vi "溶解氧电极校准.vi"() -> ()   [LabVIEW 2016, in "斯坦道多参数.lvlib"]
uses:
  <vilib>/Utility/miscctls.llb/LVPointTypeDef.ctl
  <vilib>/Analysis/NI_AALBase.lvlib
panel:
  out "标液2":string="饱和标准液"
  out "标液1":string="零点标准液"
  in  "刷新按钮":bool
  out "第二点信号值":dbl
  out "第一点信号值":dbl
  out "通讯状态":string
  out "第二点校准值":dbl
  out "第一点校准值":dbl
  out "最小值":sgl format="%#.2f"
  out "最大值":sgl format="%#.2f"
  in  "校准模式":u16(ring)=1 items=["两点校准", "单点校准"]
  in  "校准停止":bool
  in  "校准启动":bool
  out "波形图表":dbl(graph) caption="历史曲线"
  out "变异系数":dbl format="%#.6f"
  out "standard deviation":dbl caption="标准差" format="%#.2f"
  out "mean":dbl caption="均值" format="%#.2f"
  out "测量读值":dbl caption="测量值" format="%#.2f"
  out "偏移值补偿":dbl caption="溶解氧偏移修正值" format="%#.2f"
  out "饱和度值":dbl format="%#.2f"
  out "提示":string
  out "气压补偿值":dbl format="%#.2f"
  out "盐度补偿值":dbl format="%#.2f"
  out "电极斜率":dbl format="%#.6f"
  out "电极零点":dbl format="%#.6f"
  # "溶解氧电极设定"
  # "%"
  # "%"
  # "ppt"
  # "hPa"
  # "请选择校准模式:"
  # "mg/L"
  # "%"
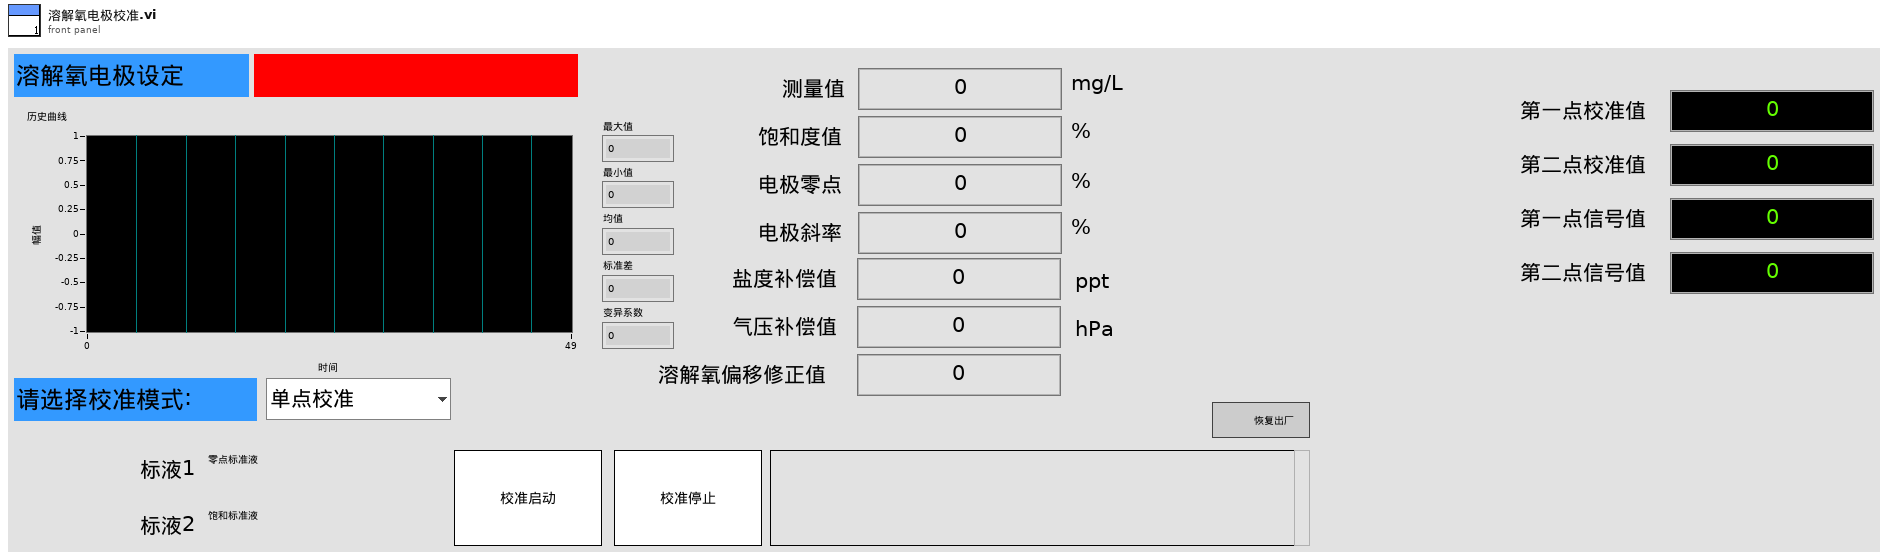
[diagram p1: front panel]
types:
  T1 = typedef "LVPointTypeDef.ctl" = cluster{"Horizontal":i16, "Vertical":i16}
  T2 = cluster{"电极状态标志":u16, "电极型号标志":u16, "溶解氧测量值":sgl, "温度测量值":sgl, "溶解氧饱和度值":sgl, "盐度补偿值":sgl, "大气压补偿值":sgl, "溶解氧偏移修正值":sgl, "温度偏移修正值":sgl, "手动温度补偿值":sgl, "溶解氧电极零点":sgl, "溶解氧电极斜率":sgl, "第1点标准值记录":sgl, "第1点信号值记录":sgl, "第1点温度值记录":sgl, "第2点标准值记录":sgl, "第2点信号值记录":sgl, "第2点温度值记录":sgl, "命令滤波设定":u16, "温度模式":enum16{"ATC", "MTC"}, "生产批次":u16, "电极序号":u16, "串口地址":u16, "串口波特率":enum16{"9600", "19200", "115200"}, "串口校验位":enum16{"NONE", "ODD", "EVEN"}, "串口停止位":enum16{"1bit", "2bit"}, "第一点标准值":sgl, "第二点标准值":sgl}
  T3 = enum8{"Enabled", "Disabled", "Disabled and Grayed Out"}
  T4 = cluster{"测量量程":dbl, "测量精度":dbl, "测量间隔":dbl, "消解温度":dbl, "消解时长":dbl, "空白校准时间":timestamp, "曲线截距":dbl, "曲线斜率":dbl, "测量检出限":dbl, "测量信号值":dbl, "线性相关系数":dbl, "二次多项式系数":dbl, "标样校准时间":timestamp, "单位":enum16{"ug/L", "mg/L"}}
  T5 = cluster{"ph":bool, "DO":bool, "Cond":bool, "Turb":bool, "叶绿素a":bool, "藻密度":bool, "ORP":bool}
  T6 = cluster{"温度测量值":sgl, "测量值":sgl, "温度偏移修正值":sgl, "信号值":sgl}
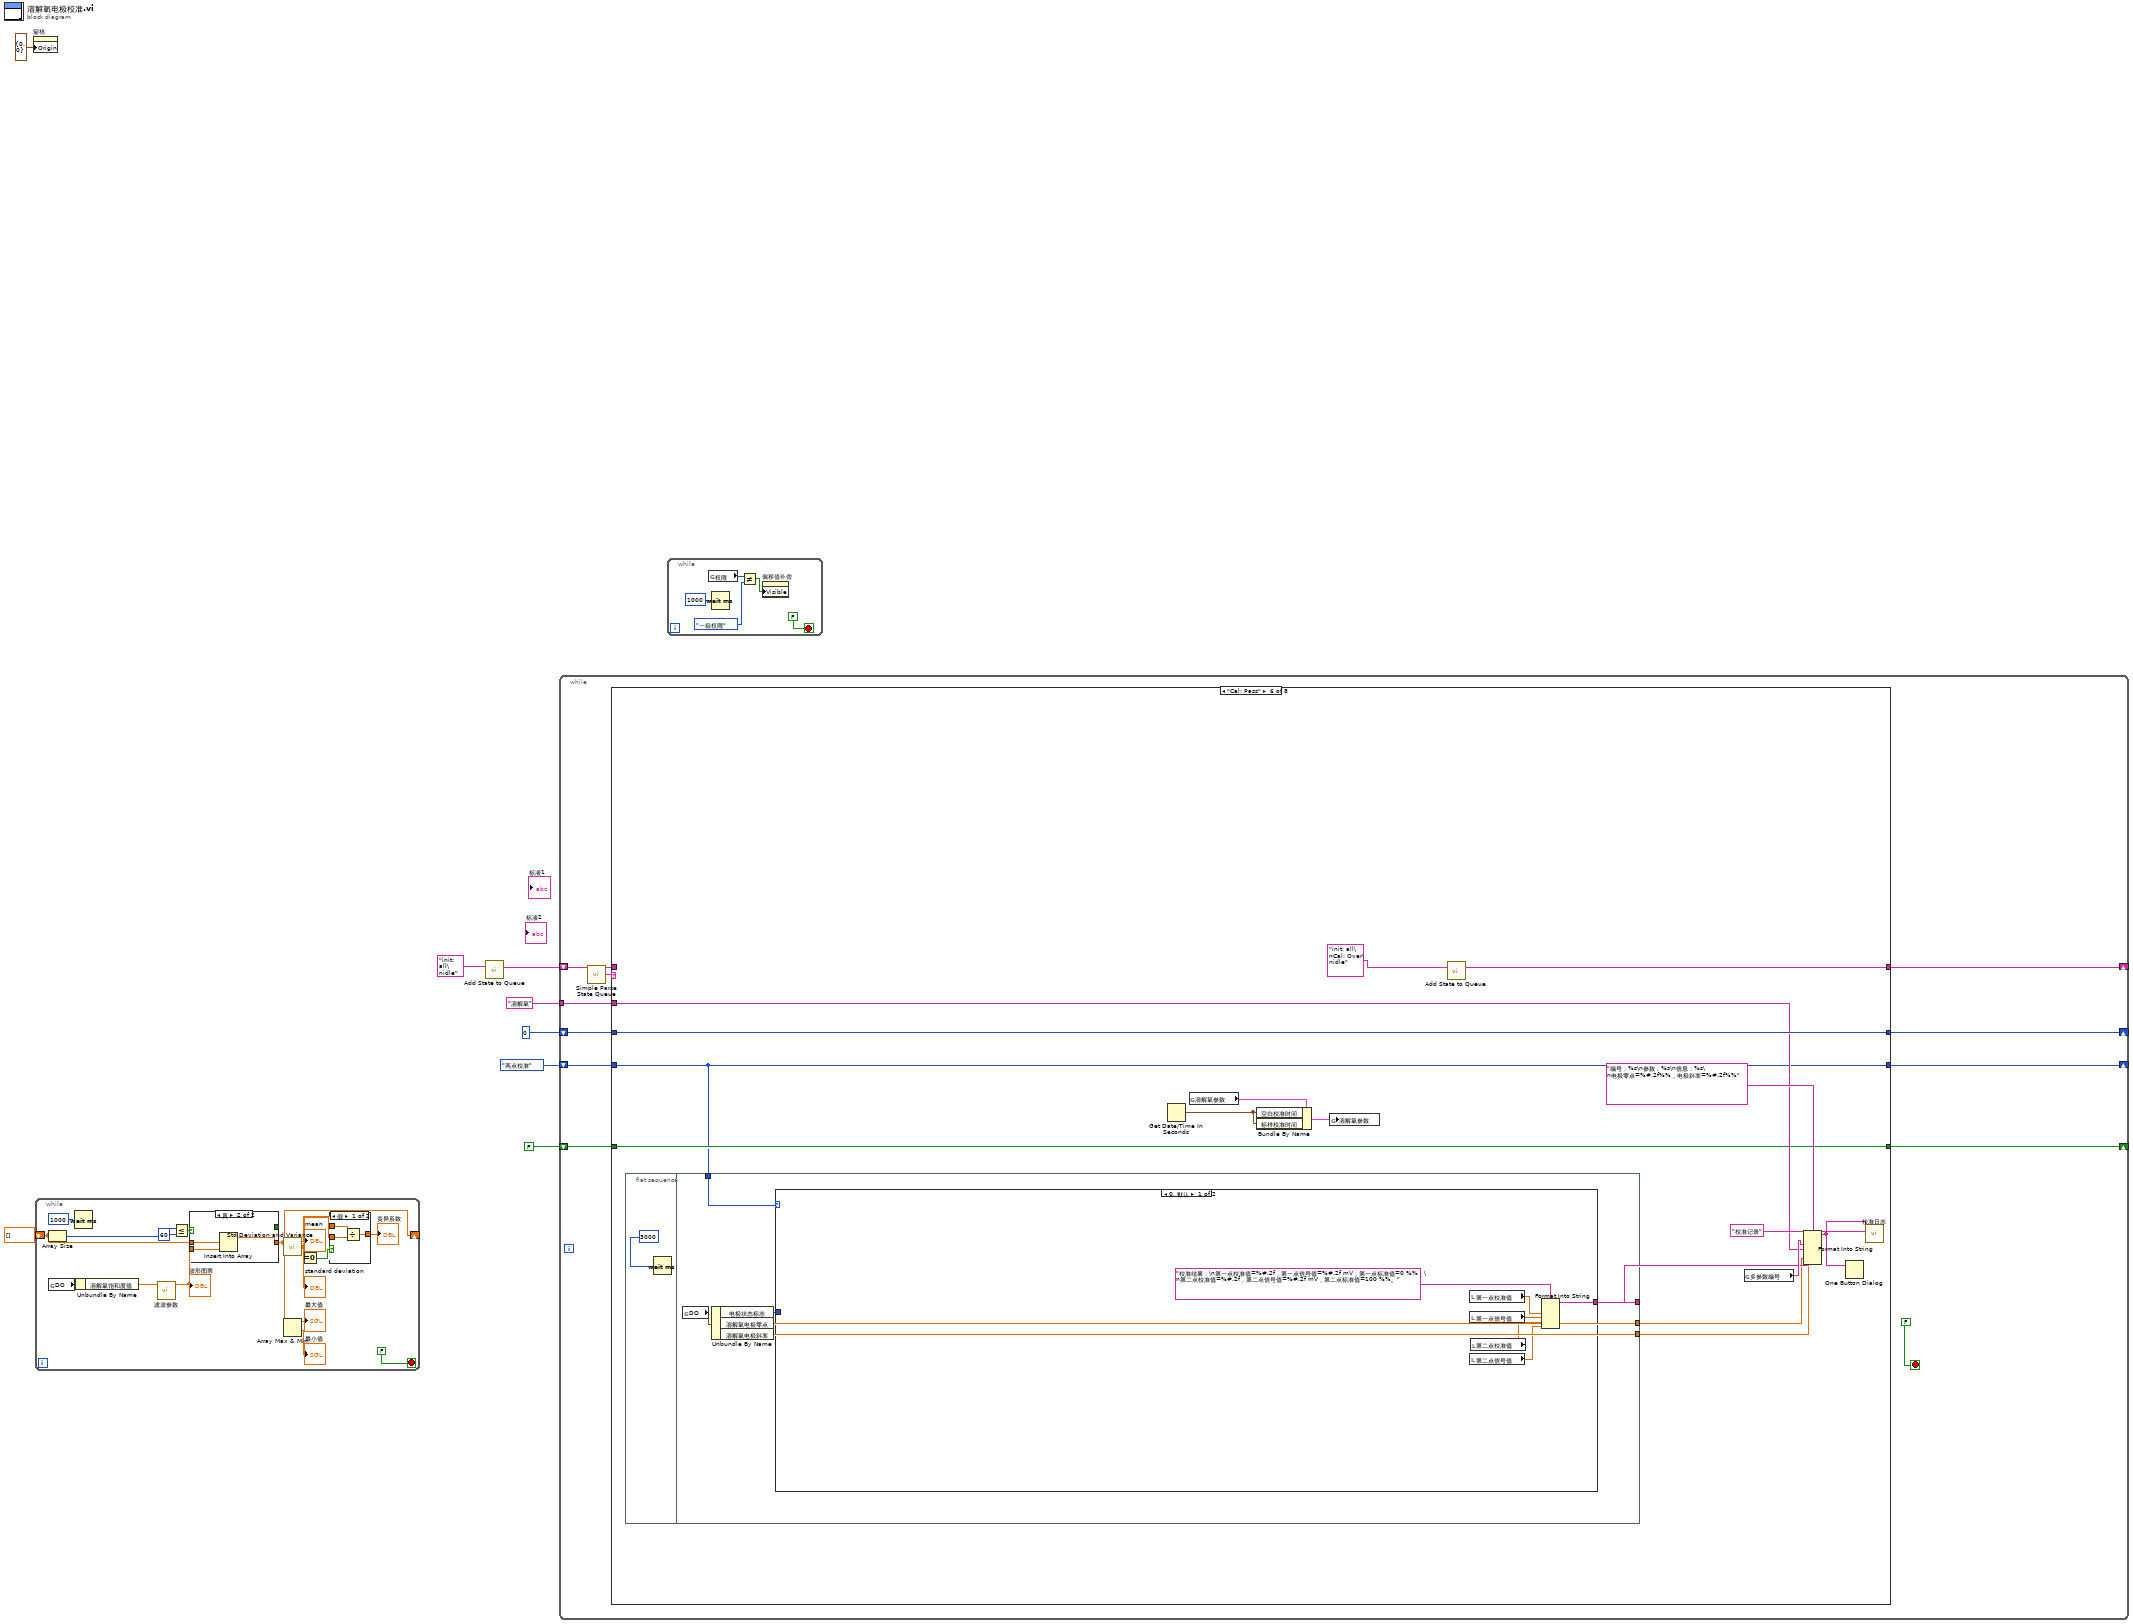
[diagram p0: block diagram]
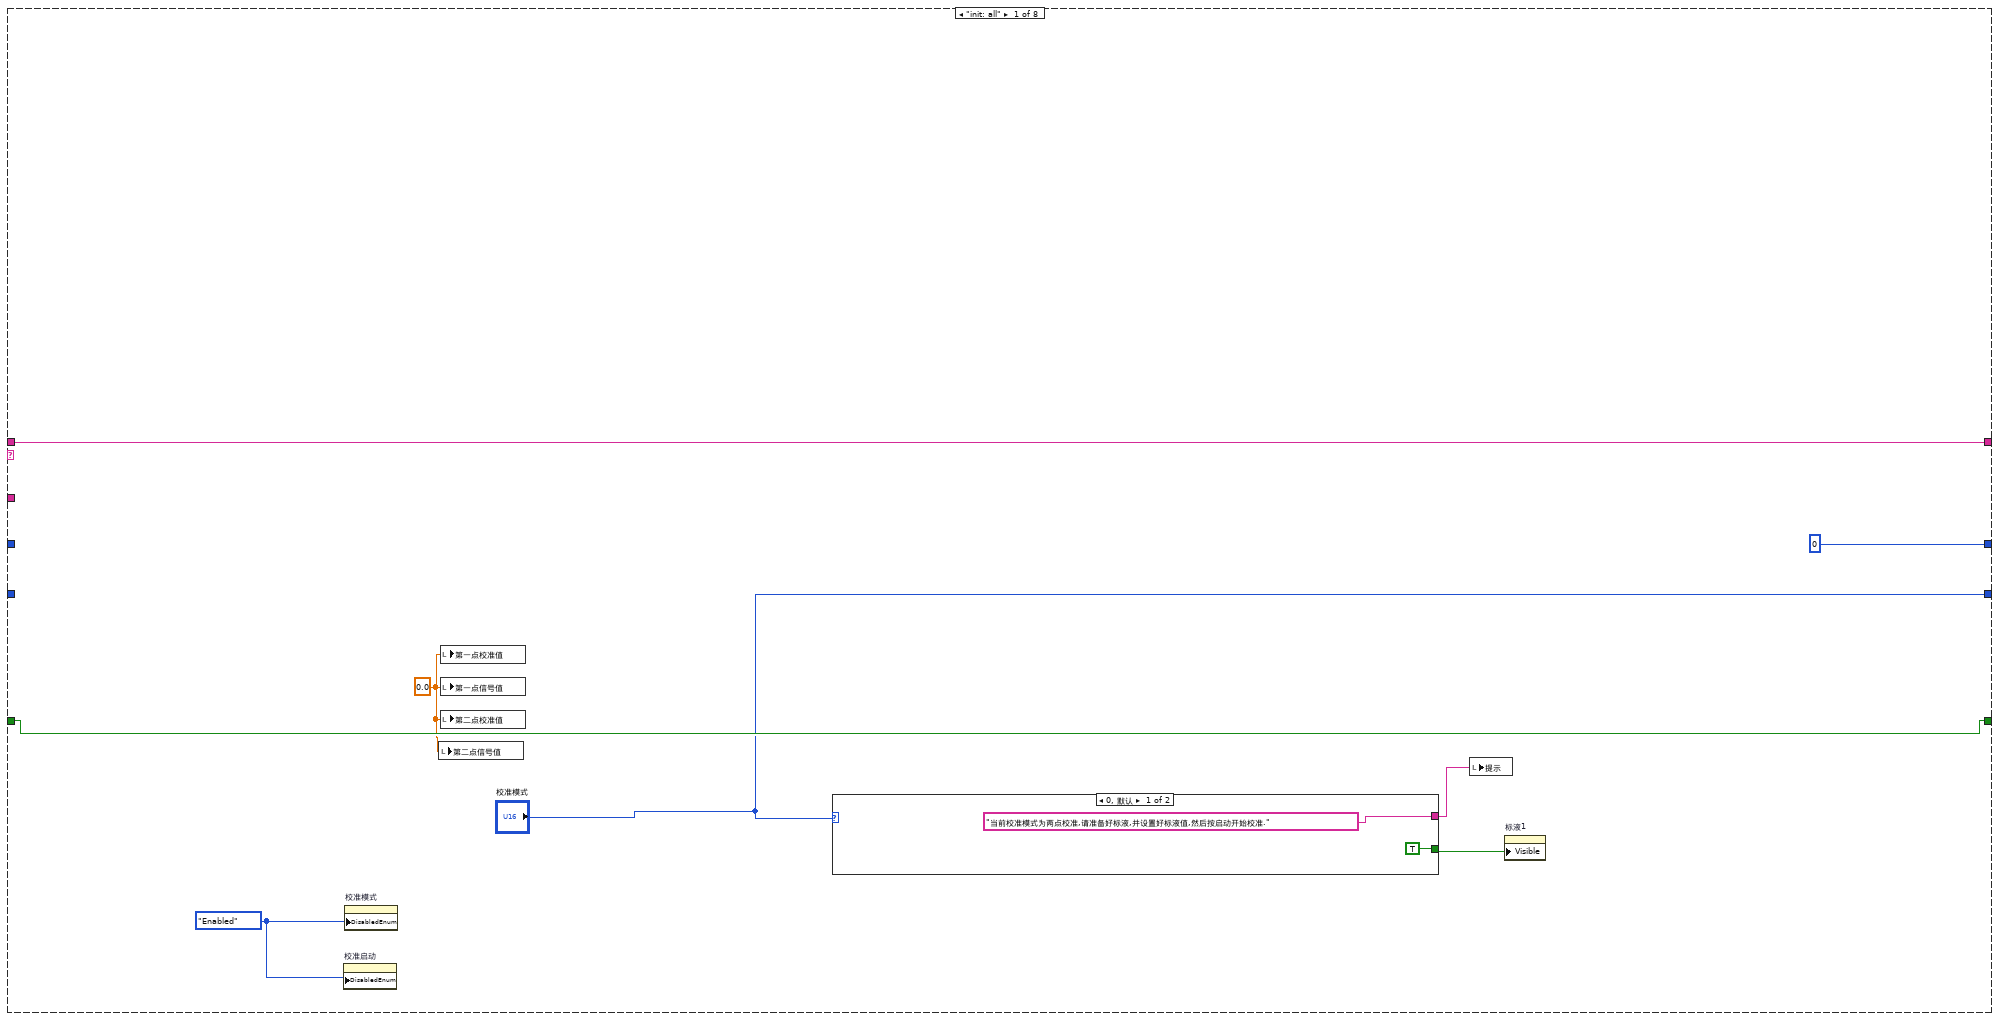
[diagram p2: hidden frame]
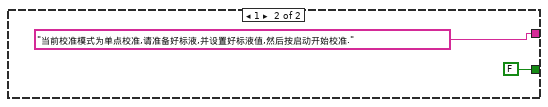
[diagram p3: hidden frame]
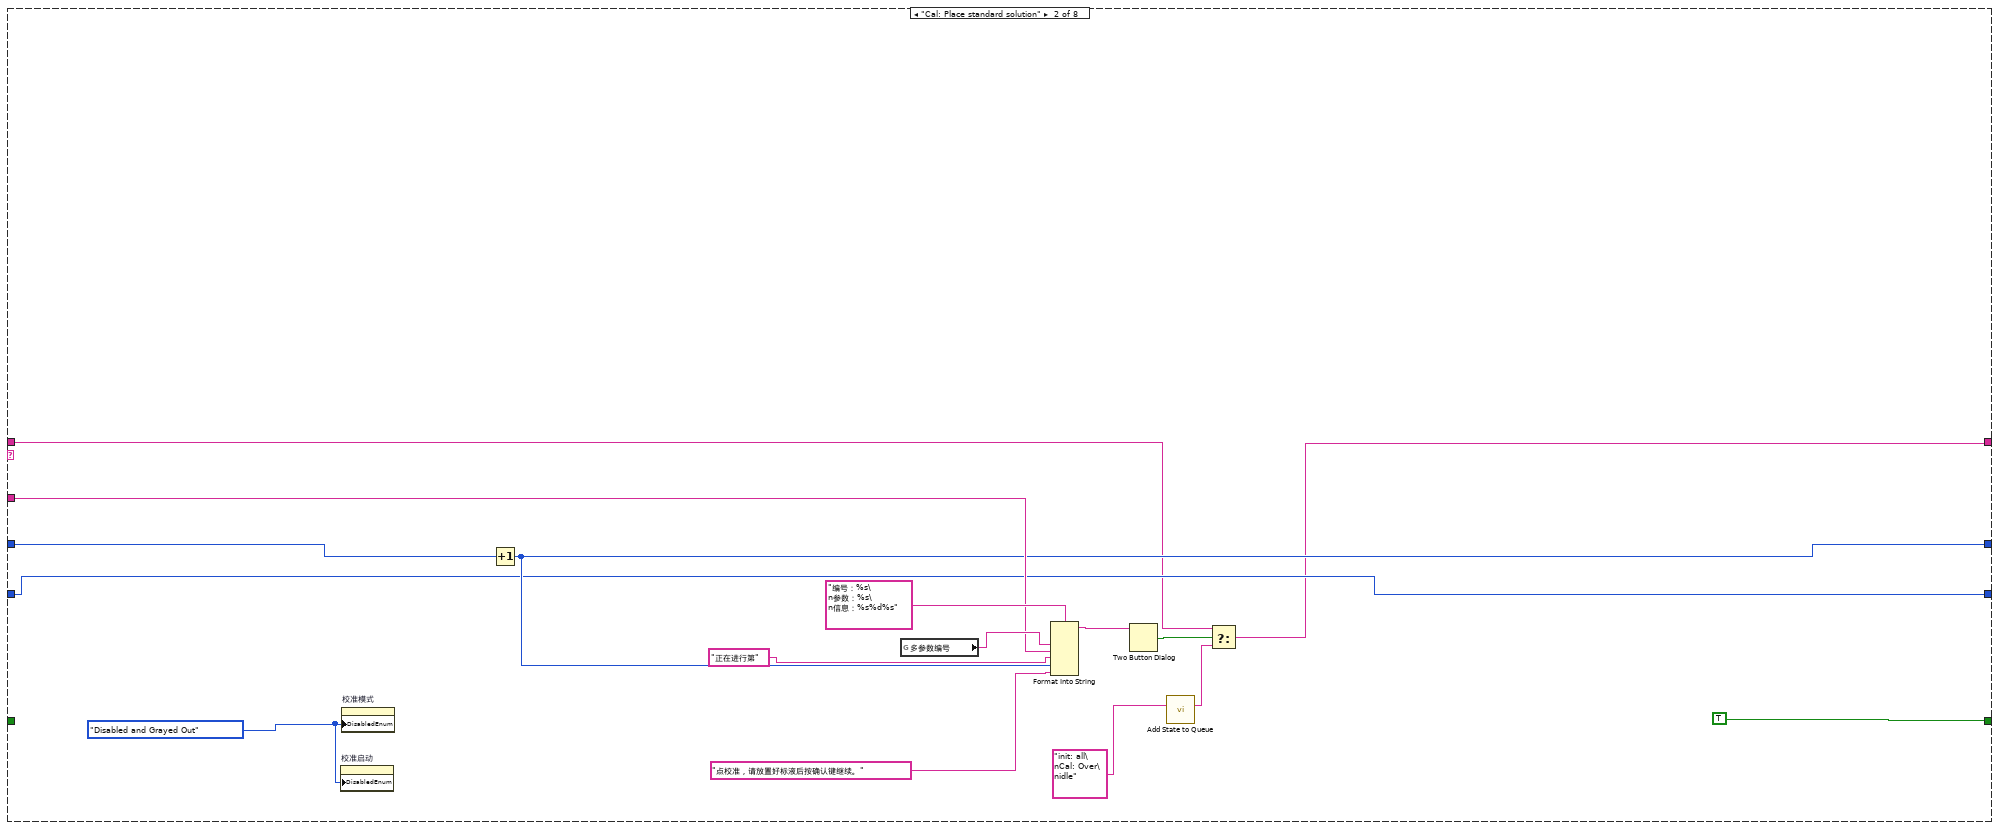
[diagram p4: hidden frame]
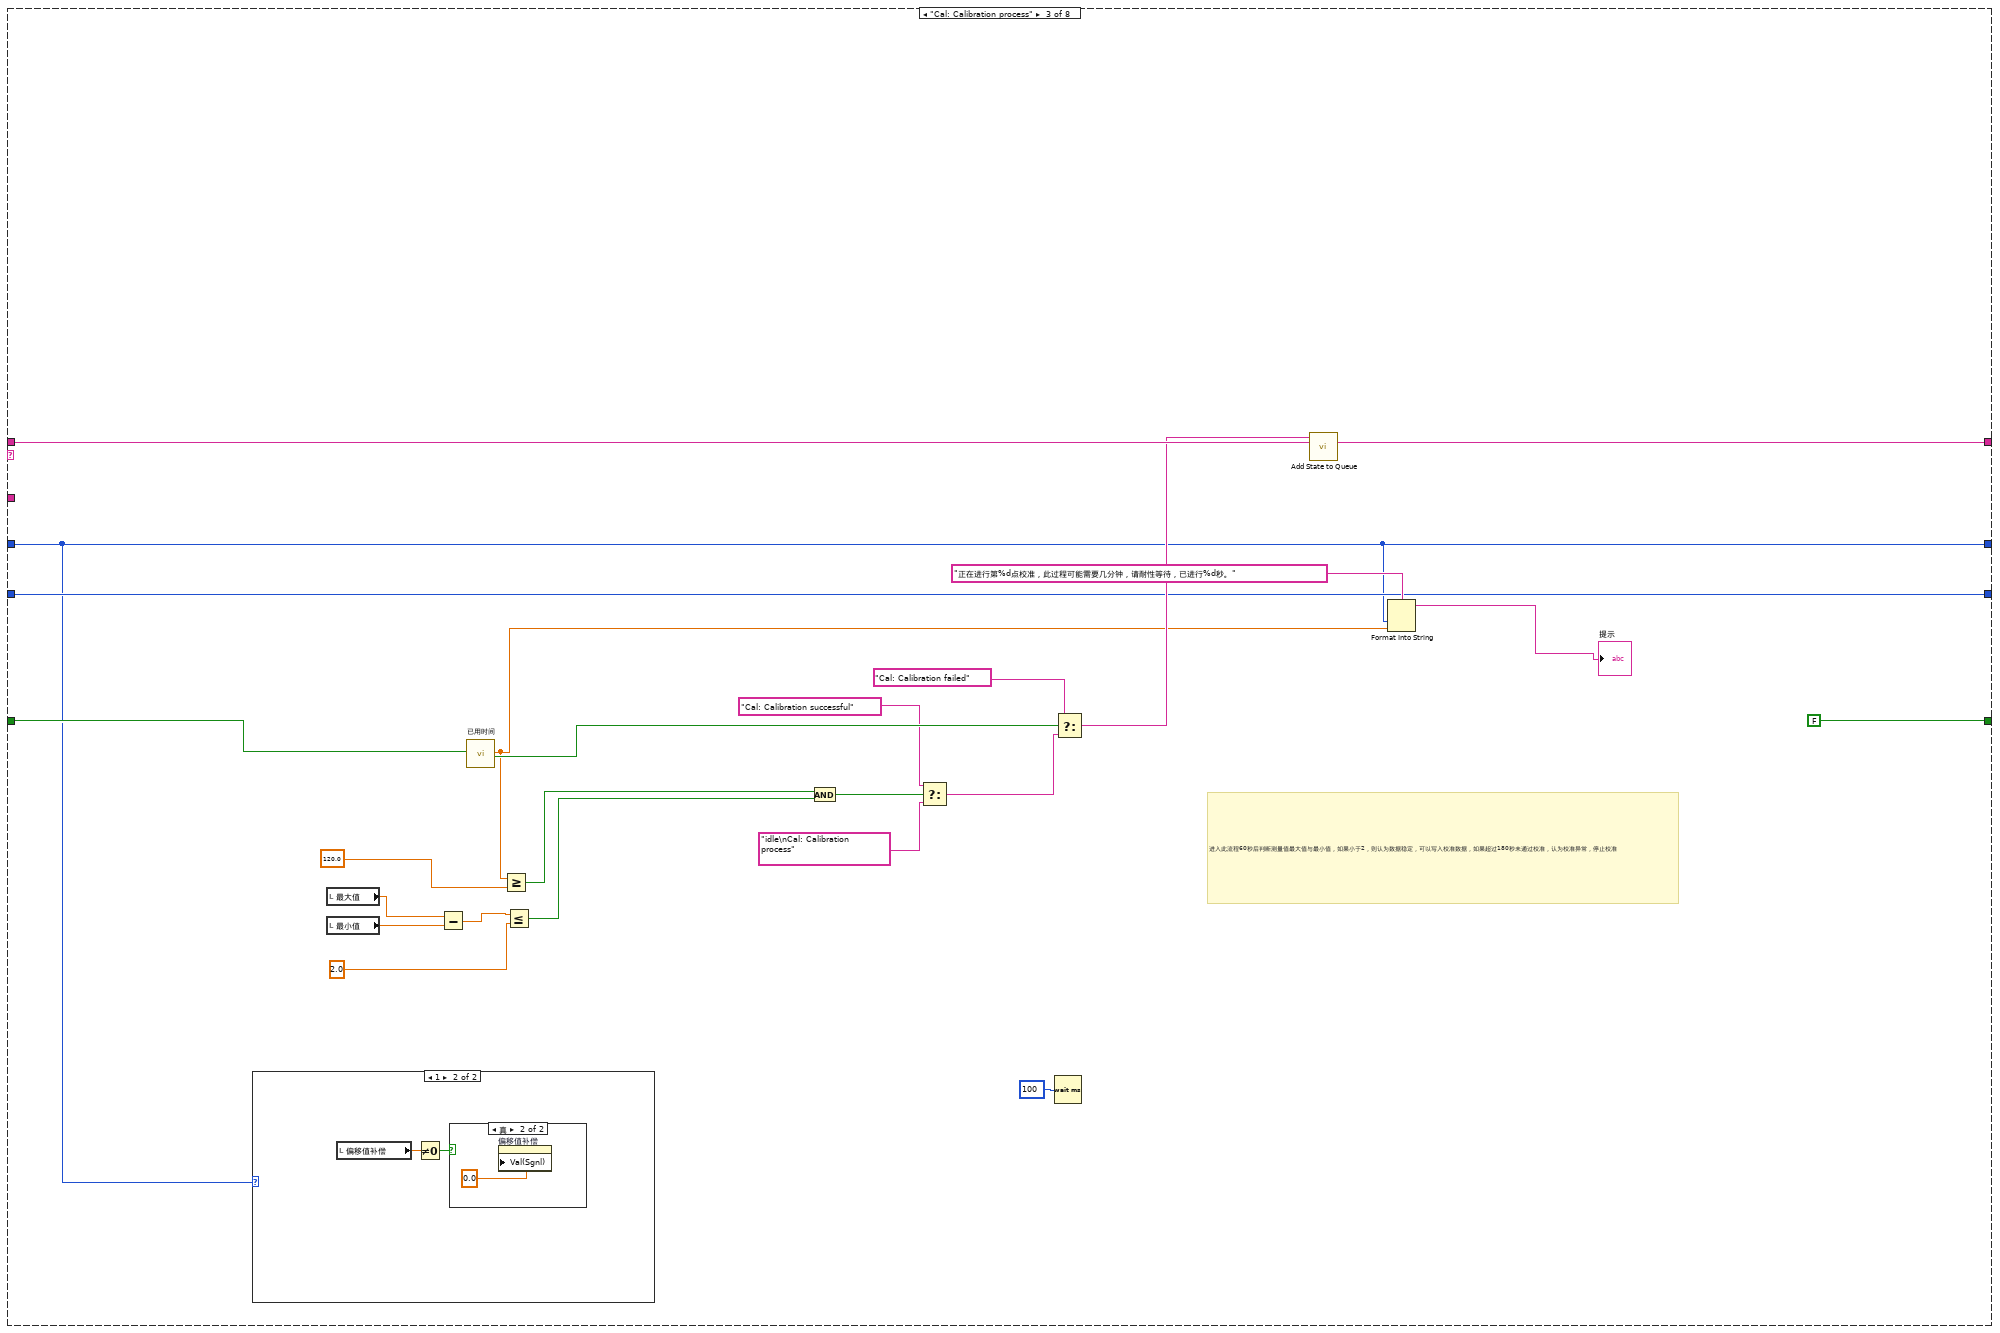
[diagram p5: hidden frame]
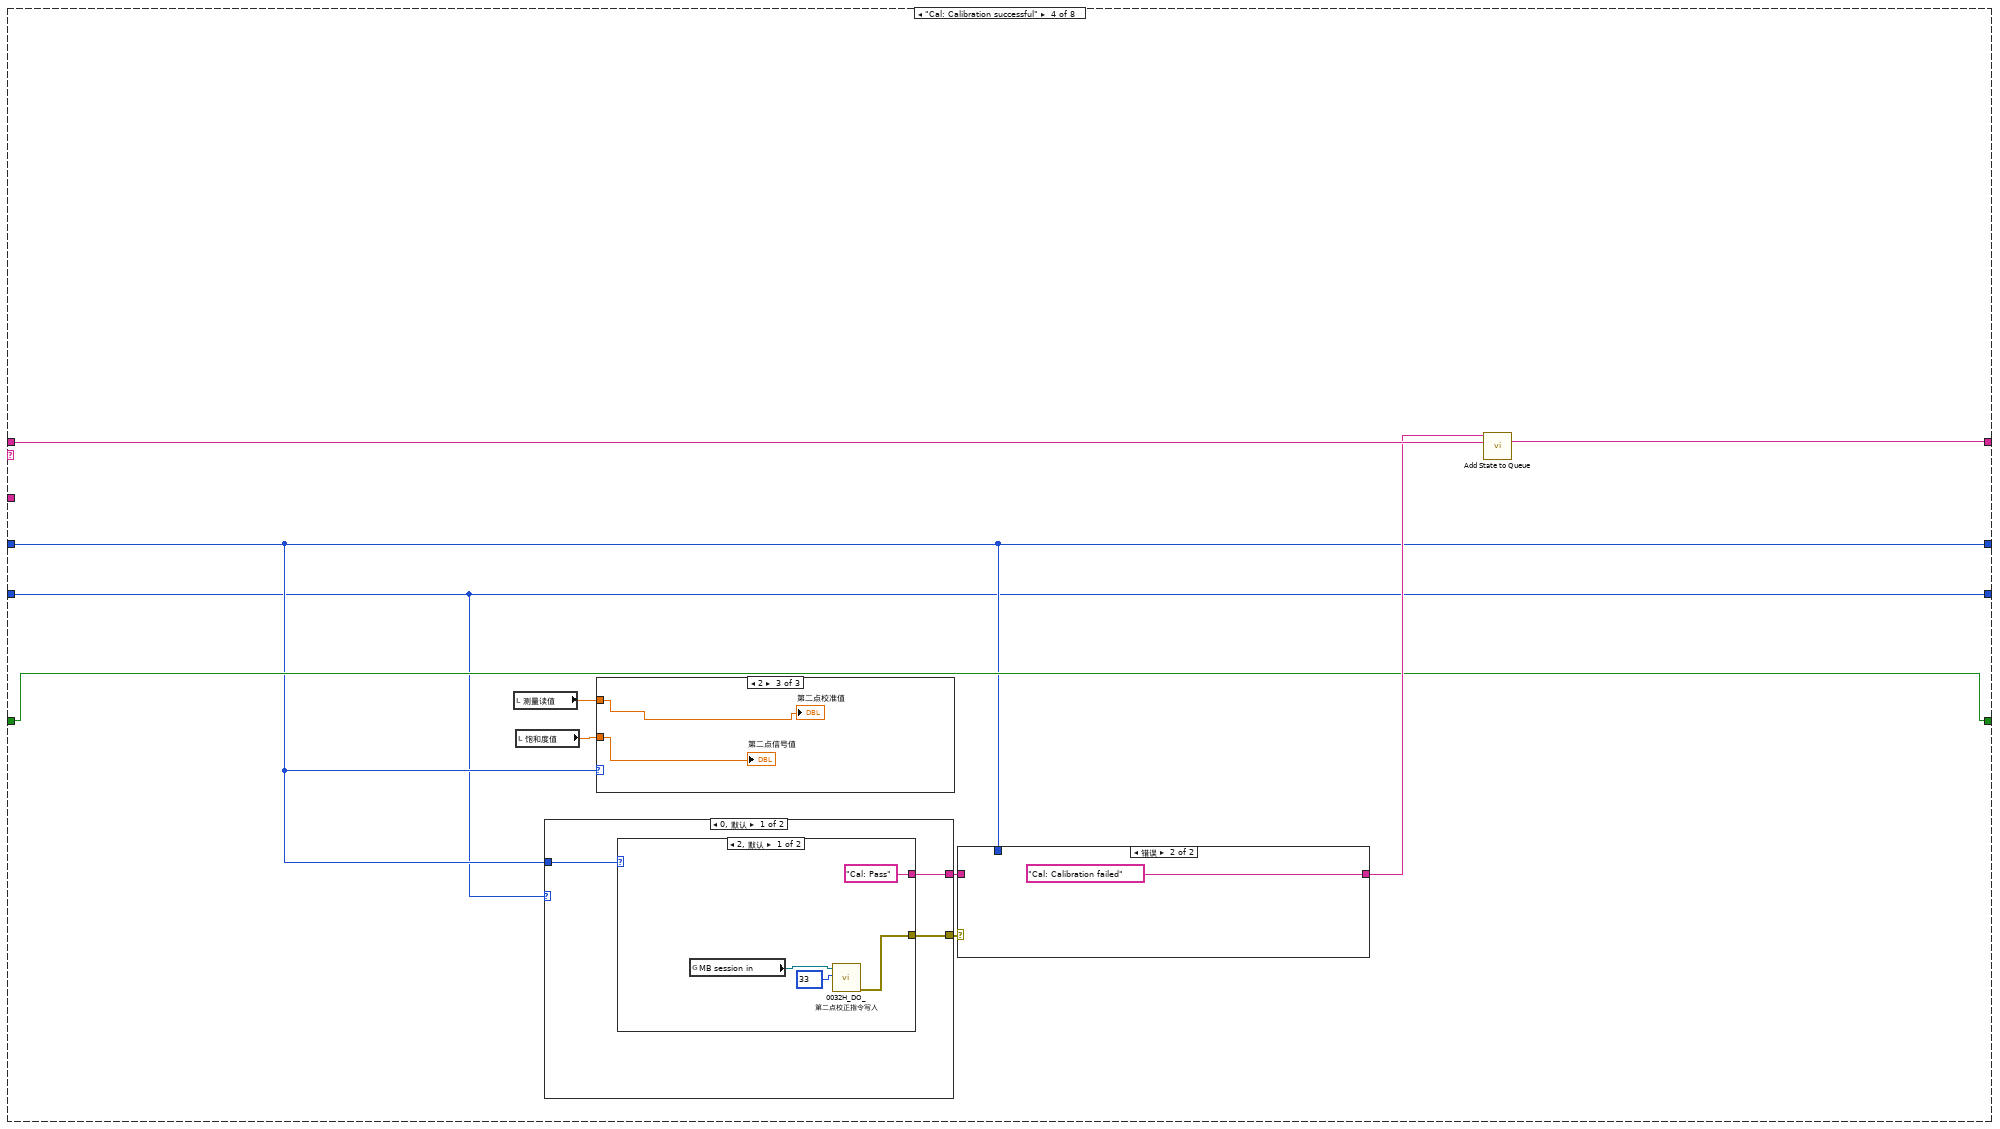
[diagram p8: hidden frame]
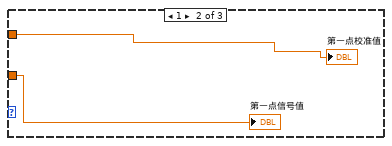
[diagram p10: hidden frame]
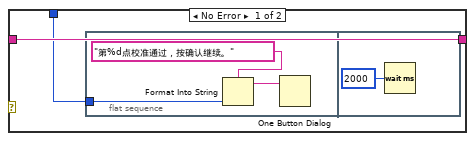
[diagram p11: hidden frame]
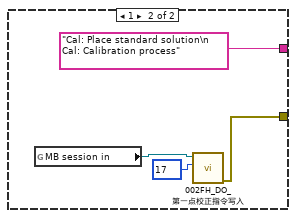
[diagram p12: hidden frame]
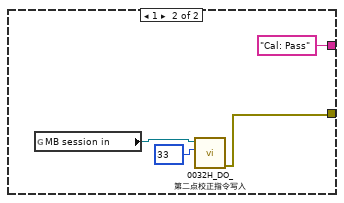
[diagram p13: hidden frame]
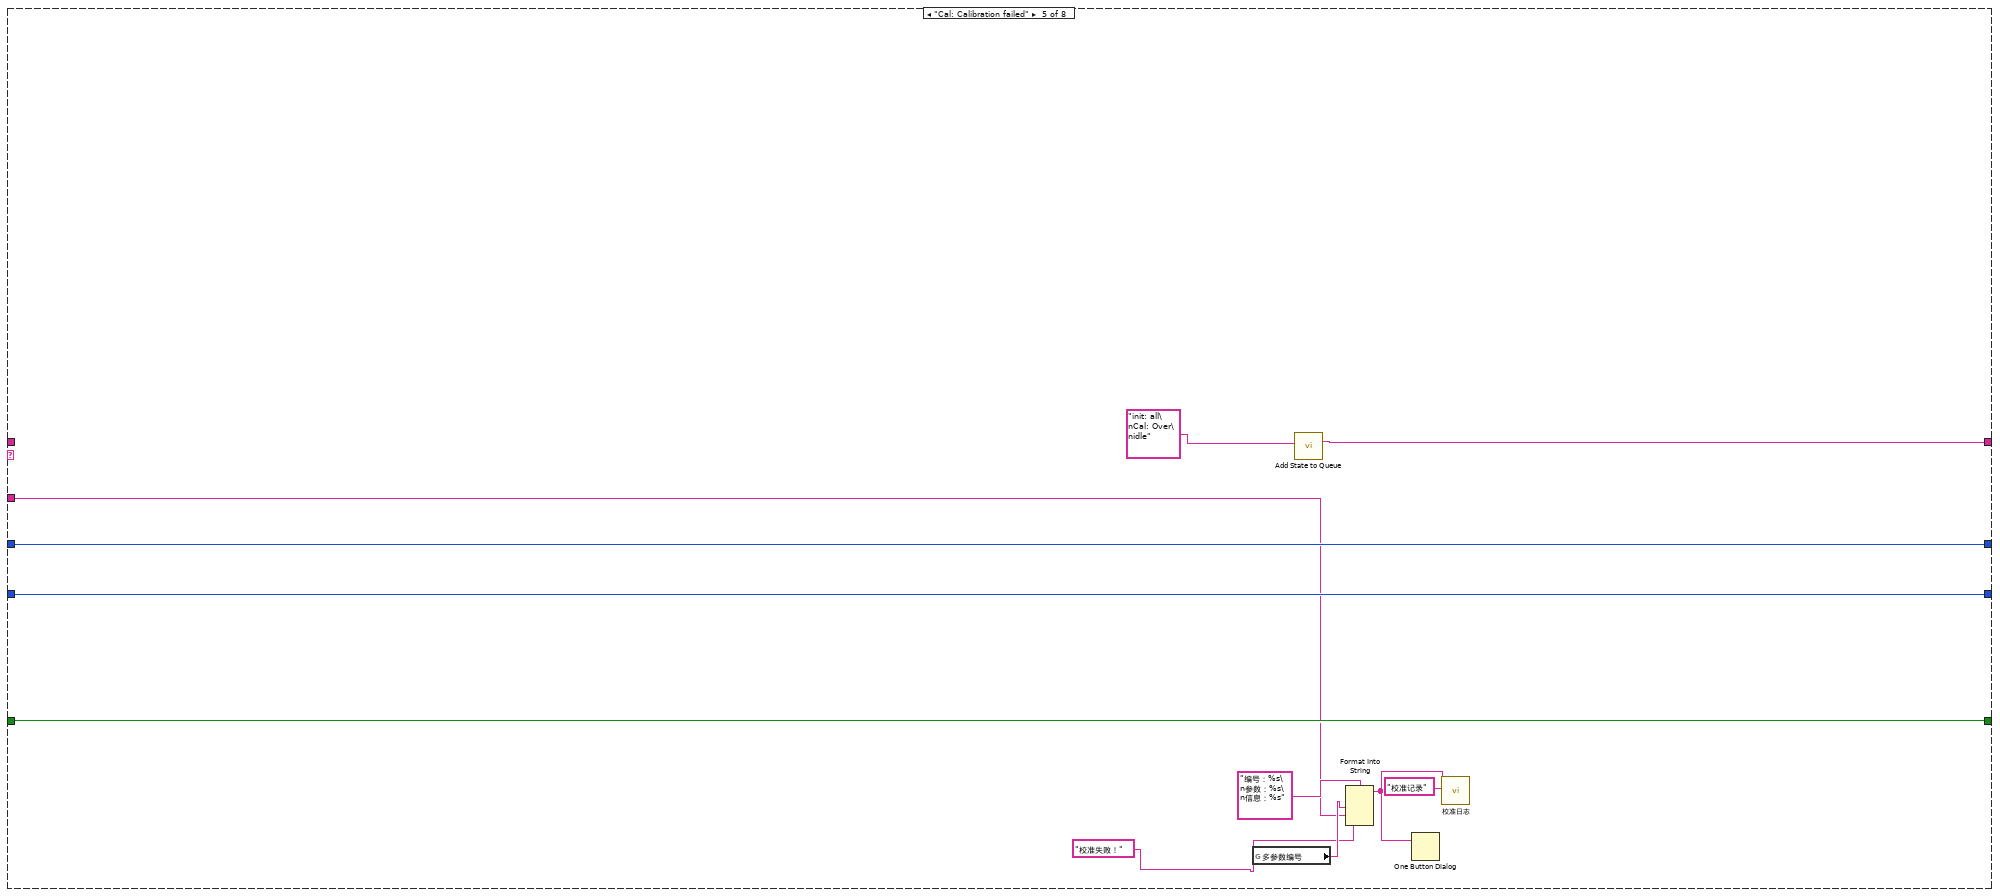
[diagram p14: hidden frame]
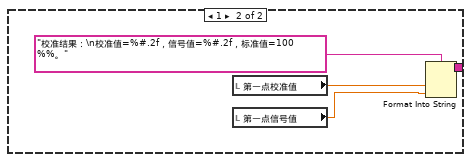
[diagram p15: hidden frame]
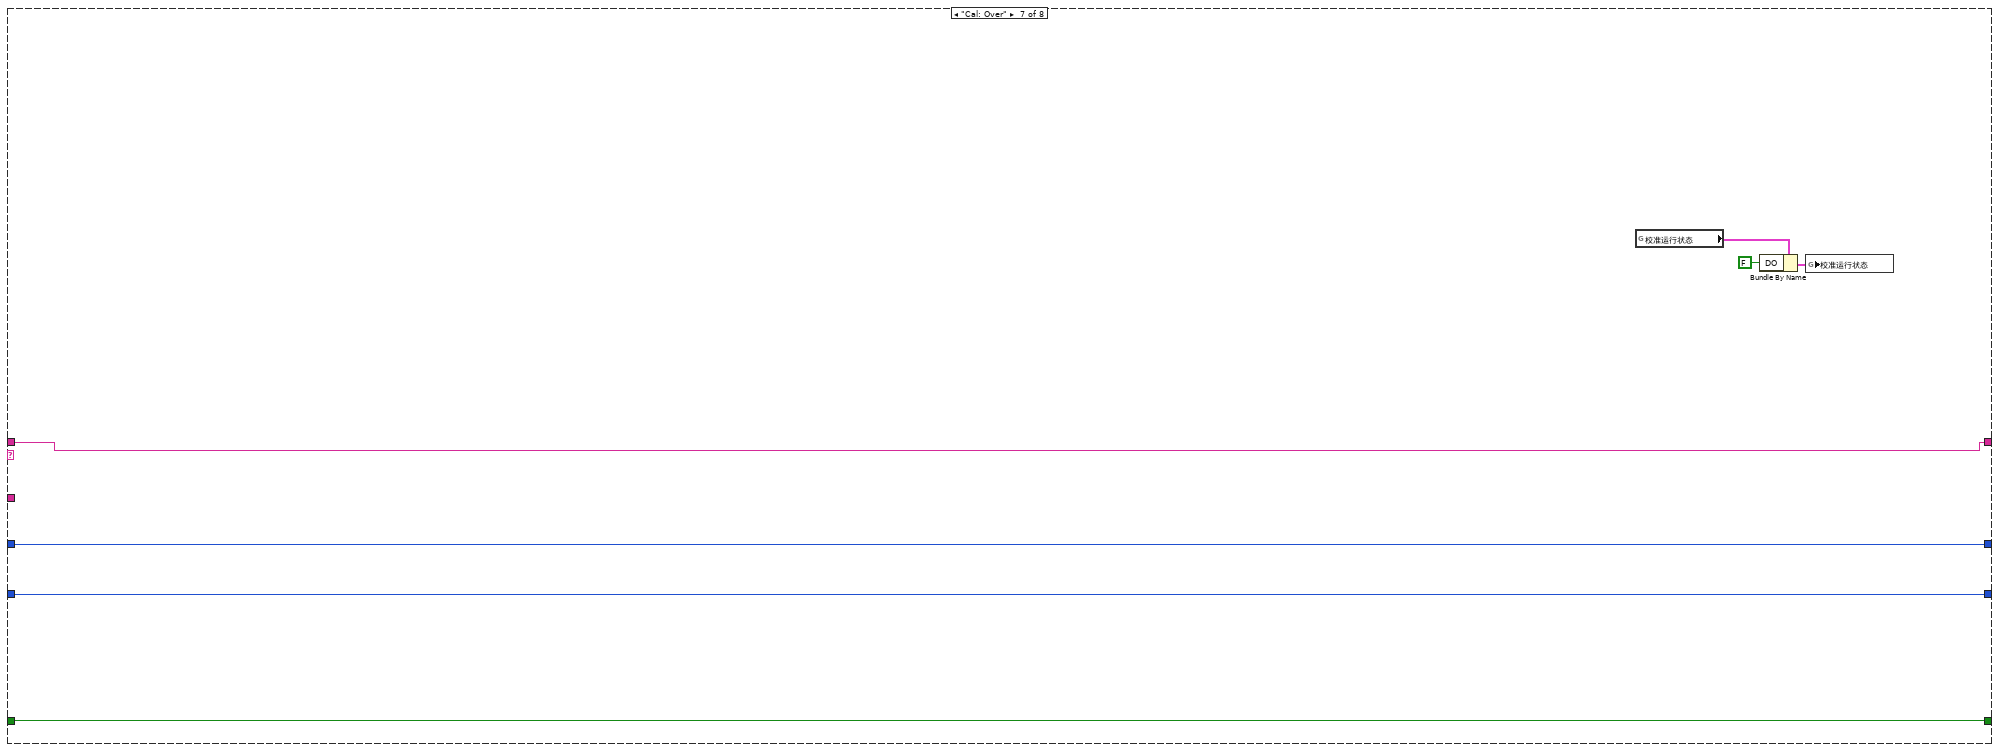
[diagram p16: hidden frame]
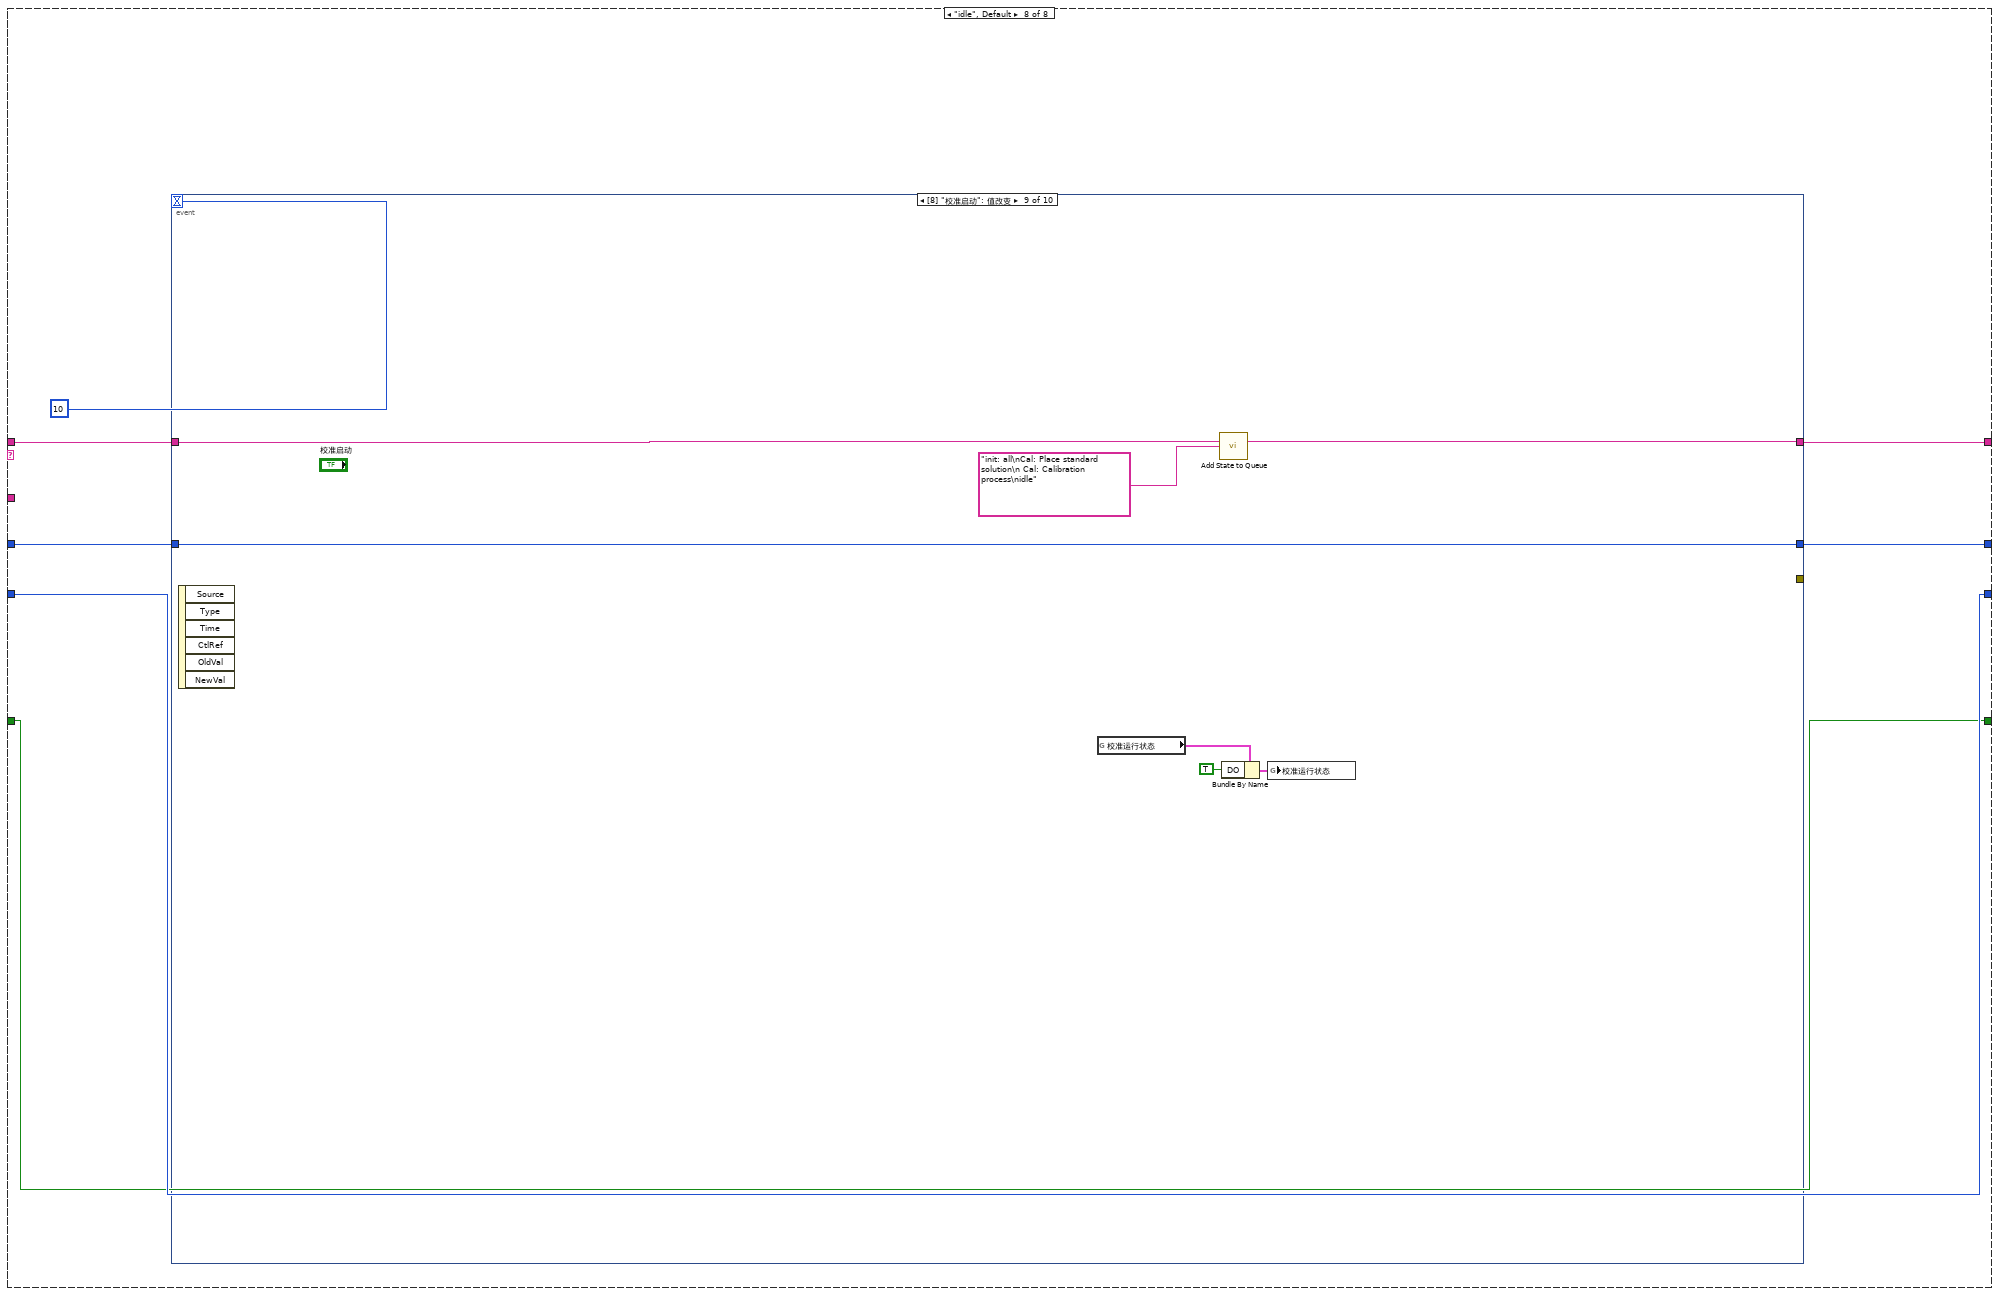
[diagram p17: hidden frame]
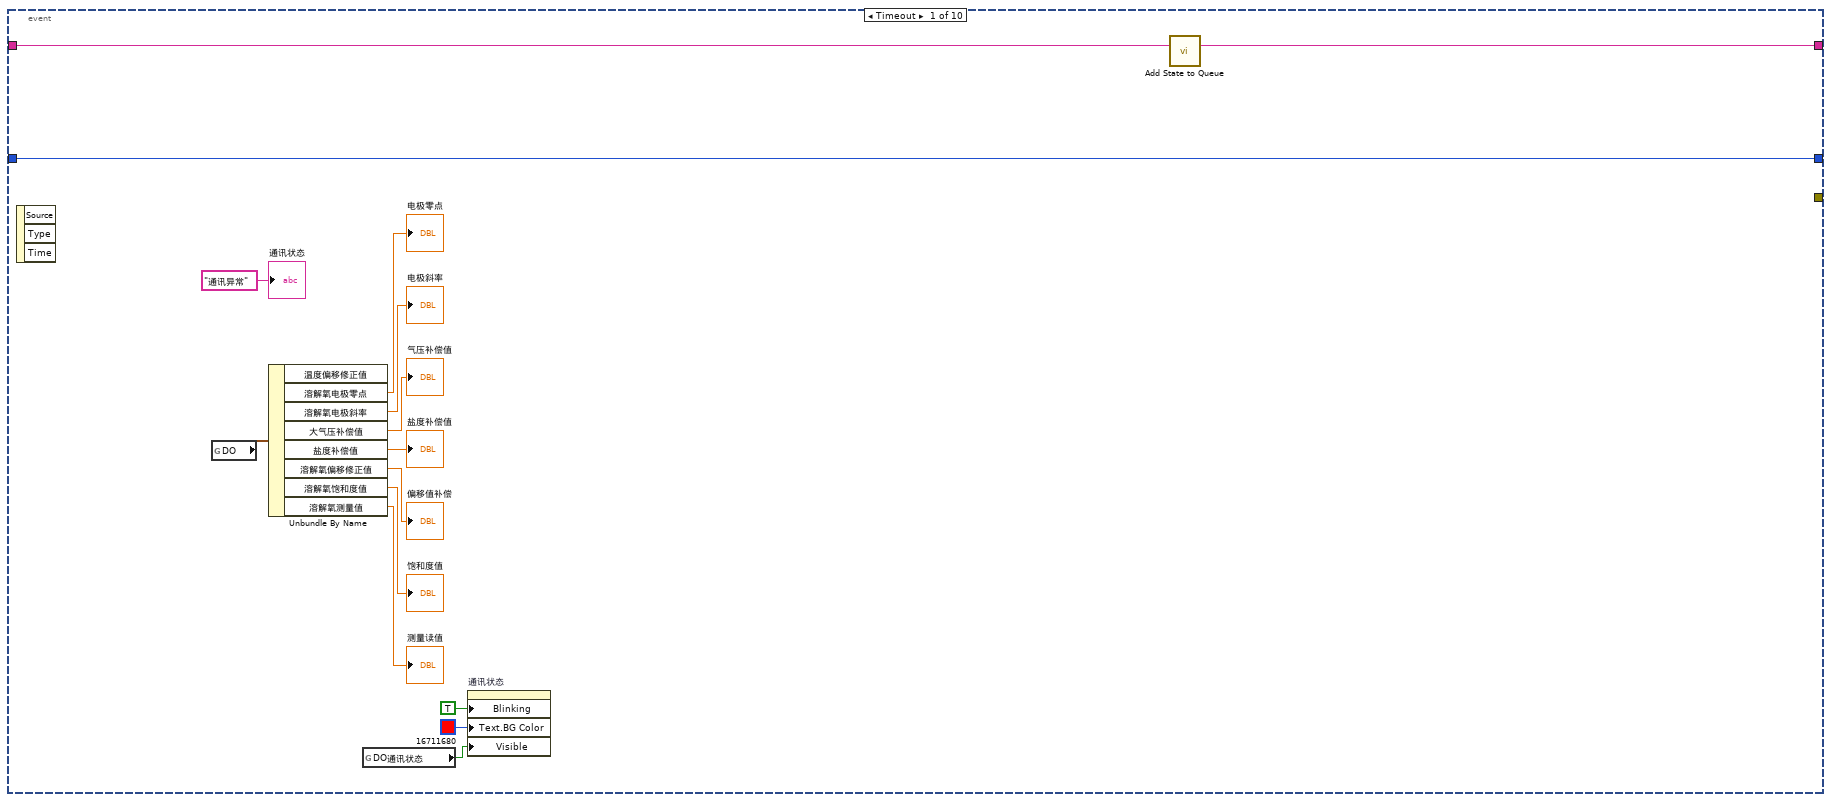
[diagram p18: hidden frame]
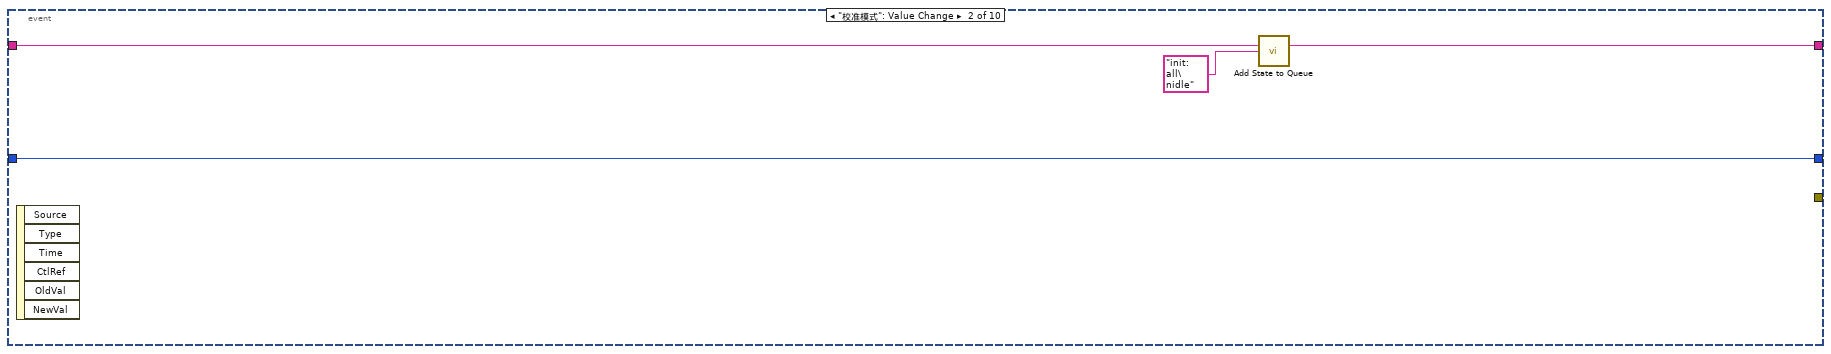
[diagram p19: hidden frame]
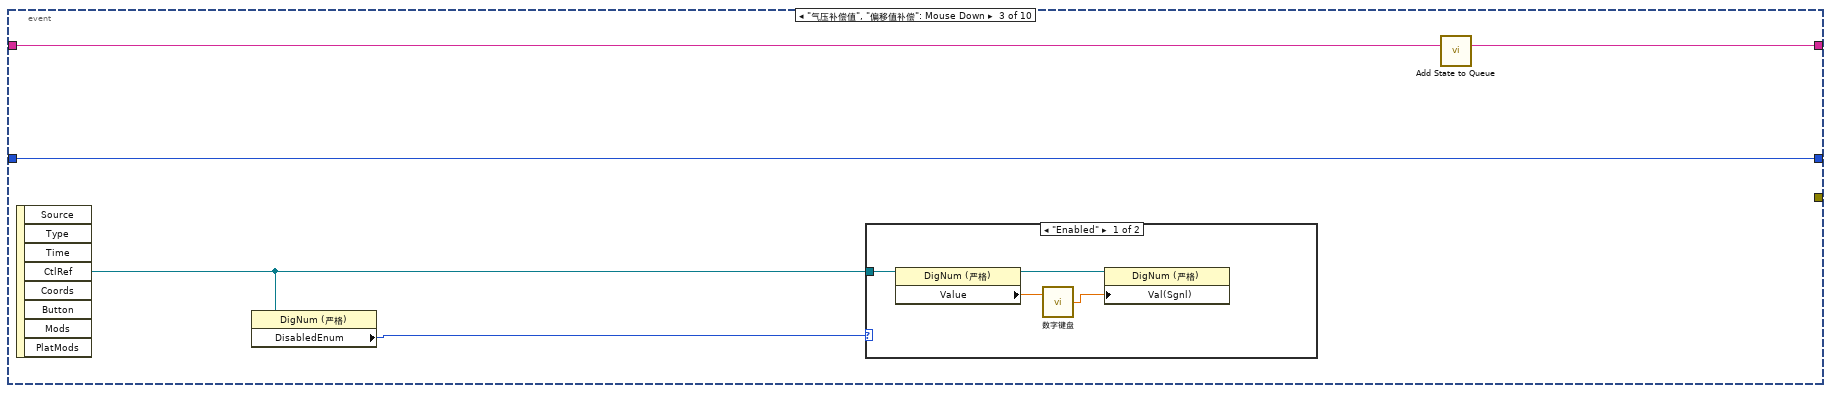
[diagram p20: hidden frame]
diagram:
  n1 = property on="窗格" class="Pane"("Origin"=T1 {"Horizontal"=0, "Vertical"=0} ("原点")) -> ()  [unwired: 2 in, 2 out]
  n2 = while {
    shift-right: [w13] -> _
    shift-left: sgl[] [] -> [w20]
    stop <- FALSE stop-if-true
    n3 = Array Size(array=w20) -> (size(s)=w22:i32)
    n4 = global read "国弘过程全局变量.vi" "DO"() -> (w16:T2)
    n5 = Wait (ms)(milliseconds to wait=u32 1000 ("等待时间（毫秒）")) -> ()  [unwired: 1 out]
    n6 = Unbundle By Name(w16) -> ("溶解氧饱和度值"=w10:sgl)
    n7 = call "滤波参数.vi"("x"=w10) -> ("mode"=w9:dbl)  [unwired: 10 in]
    "波形图表" <- w9
    n8 = Less Or Equal?(x=w22, y=60) -> (x <= y?=w21:bool)
    n9 = case shown="真" w21 {
      tunnel: w20 -> [w33 w36]
      tunnel: w9 -> [w31 w35]
      tunnel: [w29 w34] -> w13
      tunnel: [TRUE _] -> _
      frame False {
        n10 = Replace Array Subset(array=w33, new element=w31) -> (w32:sgl[])  [unwired: 1 in]
        n11 = Rotate 1D Array(1:w32, 2:-1 ("n")) -> (0:w29:sgl[])
      }
      frame True {
        n12 = Insert Into Array(array=w36, new element=w35) -> (w34:sgl[])  [unwired: 1 in]
      }
    }
    n13 = call <vilib>:"Std Deviation and Variance.vi"("X"=w13) -> ("mean"=w15:dbl, "standard deviation"=w14:dbl)  [unwired: 1 in, 1 out]
    "mean" <- w15
    "standard deviation" <- w14
    n14 = Array Max & Min(array=w13) -> (max value=→"最大值":sgl, min value=→"最小值":sgl)  [unwired: 2 out]
    n15 = Equal To 0?(x=w15) -> (x = 0?=w19:bool)
    n16 = case shown="假" w19 {
      tunnel: w14 -> [w27 _]
      tunnel: [w26 _] -> w18
      tunnel: w15 -> [w25 _]
      frame False {
        n17 = Divide(x=w27, y=w25) -> (x/y=w26:dbl)
      }
      frame True {
      }
    }
    "变异系数" <- w18
  }
  n18 = call "Add State to Queue.vi"("State(s) In (\"\")"="init: all\nidle" ("State(s) In (\"\")")) -> ("States Out"=w5:string)  [unwired: 14 in]
  n19 = while {
    shift-right: [w44] -> _
    shift-left: w5 -> [w48]
    shift-right: [w41] -> _
    shift-left: 0 -> [w43]
    tunnel: "溶解氧" ("State(s) In (\"\")") -> [w42]
    shift-right: [w39] -> _
    shift-left: enum16{"两点校准", "单点校准"}."两点校准" ("校准模式") -> [w40]
    shift-right: [w37] -> _
    shift-left: FALSE -> [w38]
    stop <- FALSE stop-if-true
    n20 = call "Simple Parse State Queue.vi"("State Queue"=w48) -> ("Remain States"=w45:string, "Next State"=w46:string)  [unwired: 13 in]
    n21 = case shown="\"Cal: Pass\"" w46 {
      tunnel: w45 -> [w56 w64 w95 w111 _ _ w190 w197]
      tunnel: [w56 w63 w94 w110 w147 w157 w190 w196] -> w44
      tunnel: w43 -> [_ w72 w79 w105 w150 w166 w189 w194]
      tunnel: w42 -> [_ w73 _ _ w141 w162 _ _]
      tunnel: [0 w70 w79 w105 w150 w166 w189 w195] -> w41
      tunnel: w40 -> [_ w69 w80 w104 w149 w158 w188 w193]
      tunnel: ["校准模式" w69 w80 w104 w149 w158 w188 w193] -> w39
      tunnel: w38 -> [w53 _ w82 w106 w148 w161 w187 w191]
      tunnel: [w53 TRUE FALSE w106 w148 w161 w187 w191] -> w37
      frame "init: all" {
        w51 = T3."Enabled" ("禁用")
        w52 = 0.0 ("第一点校准值")
        n22 = property on="校准启动" class="Bool"("DisabledEnum"=w51) -> ()  [unwired: 2 in, 2 out]
        n23 = property on="校准模式" class="Ring (严格)"("DisabledEnum"=w51) -> ()  [unwired: 2 in, 2 out]
        n24 = local write "第二点信号值"(w52) -> ()
        n25 = local write "第一点校准值"(w52) -> ()
        n26 = local write "第一点信号值"(w52) -> ()
        n27 = local write "第二点校准值"(w52) -> ()
        n28 = case shown="0, 默认" "校准模式" {
          tunnel: ["当前校准模式为两点校准,请准备好标液,并设置好标液值,然后按启动开始校准." ("提示") "当前校准模式为单点校准,请准备好标液,并设置好标液值,然后按启动开始校准." ("提示")] -> w55
          tunnel: [TRUE ("可见") FALSE ("可见")] -> w49
          frame 0, Default {
          }
          frame 1 {
          }
        }
        n29 = local write "提示"(w55) -> ()
        n30 = property on="标液1" class="Str"("Visible"=w49) -> ()  [unwired: 2 in, 2 out]
      }
      frame "Cal: Place standard solution" {
        w62 = T3."Disabled and Grayed Out" ("禁用")
        n31 = property on="校准启动" class="Bool"("DisabledEnum"=w62) -> ()  [unwired: 2 in, 2 out]
        n32 = property on="校准模式" class="Ring (严格)"("DisabledEnum"=w62) -> ()  [unwired: 2 in, 2 out]
        n33 = Increment(x=w72) -> (x+1=w70:i32)
        n34 = global read "多参数全局变量.vi" "多参数编号"() -> (w75:string)
        n35 = Format Into String(format string="编号：%s\n参数：%s\n信息：%s%d%s" ("格式字符串"), w75, w73, "正在进行第" ("消息"), w70, "点校准，请放置好标液后按确认键继续。" ("消息")) -> (resulting string=w67:string)  [unwired: 2 in, 1 out]
        n36 = Two Button Dialog(message=w67) -> (T button?=w66:bool)  [unwired: 2 in]
        n37 = call "Add State to Queue.vi"("State(s) In (\"\")"="init: all\nCal: Over\nidle" ("State(s) In (\"\")")) -> ("States Out"=w65:string)  [unwired: 14 in]
        n38 = Select(t=w64, s=w66, f=w65) -> (s? t:f=w63:string)
      }
      frame "Cal: Calibration process" {
        # "进入此流程60秒后判断测量值最大值与最小值，如果小于2，则认为数据稳定，可以写入校准数据，如果超过180秒未通过校准，认为校准异常，停止校准"
        n39 = case shown="1" w79 {
          frame 0, Default {
          }
          frame 1 {
            n40 = local read "偏移值补偿"() -> (w101:dbl)
            n41 = Not Equal To 0?(x=w101) -> (x != 0?=w102:bool)
            n42 = case shown="真" w102 {
              frame False {
              }
              frame True {
                n43 = property on="偏移值补偿" class="DigNum (严格)"("Val(Sgnl)"=0.0 ("值(信号)")) -> ()  [unwired: 2 in, 2 out]
              }
            }
          }
        }
        n44 = local read "最大值"() -> (w99:sgl)
        n45 = local read "最小值"() -> (w98:sgl)
        n46 = Subtract(x=w99, y=w98) -> (x-y=w100:sgl)
        n47 = call "已用时间"("Reset"=w82) -> ("Elapsed Time (s)"=w78:dbl, "Time has Elapsed"=w96:bool)  [unwired: 11 in, 6 out]
        n48 = Greater Or Equal?(x=w78, y=120.0) -> (x >= y?=w91:bool)
        n49 = Less Or Equal?(x=w100, y=2.0) -> (x <= y?=w87:bool)
        n50 = And(x=w91, y=w87) -> (x .and. y?=w88:bool)
        n51 = Select(t="Cal: Calibration successful" ("State(s) In (\"\")"), s=w88, f="idle\nCal: Calibration process" ("State(s) In (\"\")")) -> (s? t:f=w86:string)
        n52 = Wait (ms)(milliseconds to wait=u32 100 ("等待时间（毫秒）")) -> ()  [unwired: 1 out]
        n53 = Select(t="Cal: Calibration failed" ("State(s) In (\"\")"), s=w96, f=w86) -> (s? t:f=w85:string)
        n54 = call "Add State to Queue.vi"("State(s) In Front (\"\")"=w85, "State(s) In (\"\")"=w95) -> ("States Out"=w94:string)  [unwired: 13 in]
        n55 = Format Into String(format string="正在进行第%d点校准，此过程可能需要几分钟，请耐性等待，已进行%d秒。" ("格式字符串"), w79, w78) -> (resulting string=→"提示":string)  [unwired: 2 in, 1 out]
      }
      frame "Cal: Calibration successful" {
        n56 = local read "测量读值"() -> (w107:dbl)
        n57 = local read "饱和度值"() -> (w108:dbl)
        n58 = case shown="0, 默认" w104 {
          tunnel: [w127 w136] -> w113
          tunnel: [w126 "Cal: Pass" ("State(s) In (\"\")")] -> w112
          tunnel: w105 -> [w125 _]
          frame 0, Default {
            n59 = case shown="2, 默认" w125 {
              tunnel: [w128 w132] -> w127
              tunnel: ["Cal: Pass" ("State(s) In (\"\")") "Cal: Place standard solution\n Cal: Calibration process" ("State(s) In (\"\")")] -> w126
              frame 2, Default {
                n60 = global read "多参数全局变量.vi" "MB session in"() -> (w129:refnum<class "MB_Master.lvclass">)
                n61 = call "0032H_DO_第二点校正指令写入.vi"("数值"=u16 33, "MB session in"=w129) -> ("error out"=w128:errorcluster)  [unwired: 8 in, 1 out]
              }
              frame 1 {
                n62 = global read "多参数全局变量.vi" "MB session in"() -> (w133:refnum<class "MB_Master.lvclass">)
                n63 = call "002FH_DO_第一点校正指令写入.vi"("数值"=u16 17, "MB session in"=w133) -> ("error out"=w132:errorcluster)  [unwired: 8 in, 1 out]
              }
            }
          }
          frame 1 {
            n64 = global read "多参数全局变量.vi" "MB session in"() -> (w138:refnum<class "MB_Master.lvclass">)
            n65 = call "0032H_DO_第二点校正指令写入.vi"("数值"=u16 33, "MB session in"=w138) -> ("error out"=w136:errorcluster)  [unwired: 8 in, 1 out]
          }
        }
        n66 = case shown="2" w105 {
          tunnel: w108 -> [_ w115 w117]
          tunnel: w107 -> [_ w114 w116]
          frame 0, Default {
          }
          frame 1 {
            "第一点信号值" <- w115
            "第一点校准值" <- w114
          }
          frame 2 {
            "第二点信号值" <- w117
            "第二点校准值" <- w116
          }
        }
        n67 = case shown="错误" w113 {
          tunnel: w112 -> [w119 _]
          tunnel: [w119 "Cal: Calibration failed" ("State(s) In (\"\")")] -> w109
          tunnel: w105 -> [w118 _]
          frame No Error {
            n68 = flat-sequence {
              tunnel: w118 -> [w120]
              frame #0 {
                n69 = Format Into String(format string="第%d点校准通过，按确认继续。" ("格式字符串"), w120) -> (resulting string=w122:string)  [unwired: 2 in, 1 out]
                n70 = One Button Dialog(message=w122) -> ()  [unwired: 1 in, 1 out]
              }
              frame #1 {
                n71 = Wait (ms)(milliseconds to wait=u32 2000 ("等待时间（毫秒）")) -> ()  [unwired: 1 out]
              }
            }
          }
          frame Error {
          }
        }
        n72 = call "Add State to Queue.vi"("State(s) In Front (\"\")"=w109, "State(s) In (\"\")"=w111) -> ("States Out"=w110:string)  [unwired: 13 in]
      }
      frame "Cal: Calibration failed" {
        n73 = global read "多参数全局变量.vi" "多参数编号"() -> (w144:string)
        n74 = call "Add State to Queue.vi"("State(s) In (\"\")"="init: all\nCal: Over\nidle" ("State(s) In (\"\")")) -> ("States Out"=w147:string)  [unwired: 14 in]
        n75 = Format Into String(format string="编号：%s\n参数：%s\n信息：%s" ("格式字符串"), w144, w141, "校准失败！" ("消息")) -> (resulting string=w143:string)  [unwired: 2 in, 1 out]
        n76 = One Button Dialog(message=w143) -> ()  [unwired: 1 in, 1 out]
        n77 = call "校准日志.vi"("table"="校准记录", "日志信息"=w143) -> ()  [unwired: 9 in, 1 out]
      }
      frame "Cal: Pass" {
        n78 = flat-sequence {
          tunnel: [w171] -> w159
          tunnel: w158 -> [w170]
          tunnel: [w169] -> w156
          tunnel: [w168] -> w155
          frame #0 {
            n79 = Wait (ms)(milliseconds to wait=u32 3000 ("等待时间（毫秒）")) -> ()  [unwired: 1 out]
          }
          frame #1 {
            n80 = global read "国弘过程全局变量.vi" "DO"() -> (w172:T2)
            n81 = Unbundle By Name(w172) -> ("电极状态标志"=w173:u16, "溶解氧电极零点"=w169:sgl, "溶解氧电极斜率"=w168:sgl)
            n82 = case shown="0, 默认" w170 {
              tunnel: [w179 w183] -> w171
              tunnel: w173 -> [_ _]
              frame 0, Default {
                n83 = local read "第一点校准值"() -> (w177:dbl)
                n84 = local read "第一点信号值"() -> (w178:dbl)
                n85 = local read "第二点信号值"() -> (w174:dbl)
                n86 = local read "第二点校准值"() -> (w175:dbl)
                n87 = Format Into String(format string="校准结果：\n第一点校准值=%#.2f，第一点信号值=%#.2f mV，第一点标准值=0 %%；\n第二点校准值=%#.2f，第二点信号值=%#.2f mV，第二点标准值=100 %%。" ("提示"), w177, w178, w175, w174) -> (resulting string=w179:string)  [unwired: 2 in, 1 out]
              }
              frame 1 {
                n88 = local read "第一点校准值"() -> (w182:dbl)
                n89 = local read "第一点信号值"() -> (w180:dbl)
                n90 = Format Into String(format string="校准结果：\n校准值=%#.2f，信号值=%#.2f，标准值=100 %%。" ("提示"), w182, w180) -> (resulting string=w183:string)  [unwired: 2 in, 1 out]
              }
            }
          }
        }
        n91 = Get Date/Time In Seconds() -> (seconds since 1Jan1904=w151:timestamp)
        n92 = global read "断电保存变量.vi" "溶解氧参数"() -> (w153:T4)
        n93 = Bundle By Name(cluster=w153, "空白校准时间"=w151, "标样校准时间"=w151) -> (w152:T4)
        n94 = global write "断电保存变量.vi" "溶解氧参数"(w152) -> ()
        n95 = call "Add State to Queue.vi"("State(s) In (\"\")"="init: all\nCal: Over\nidle" ("State(s) In (\"\")")) -> ("States Out"=w157:string)  [unwired: 14 in]
        n96 = global read "多参数全局变量.vi" "多参数编号"() -> (w163:string)
        n97 = Format Into String(format string="编号：%s\n参数：%s\n信息：%s\n电极零点=%#.2f%%，电极斜率=%#.2f%%" ("格式字符串"), w163, w162, w159, w156, w155) -> (resulting string=w160:string)  [unwired: 2 in, 1 out]
        n98 = One Button Dialog(message=w160) -> ()  [unwired: 1 in, 1 out]
        n99 = call "校准日志.vi"("table"="校准记录", "日志信息"=w160) -> ()  [unwired: 9 in, 1 out]
      }
      frame "Cal: Over" {
        n100 = global read "多参数全局变量.vi" "校准运行状态"() -> (w185:T5)
        n101 = Bundle By Name(cluster=w185, "DO"=FALSE) -> (w186:T5)
        n102 = global write "多参数全局变量.vi" "校准运行状态"(w186) -> ()
      }
      frame "idle", Default {
        n103 = event shown="[8] \"校准启动\": 值改变" {
          selector: _ -> [_ _ _ _ _ _ _ _ _ _]
          dyn-events: _ -> [_ _ _ _ _ _ _ _ _ _]
          timeout: 10 -> [_ _ _ _ _ _ _ _ _ _]
          tunnel: [_ _ _ _ w243 w249 w255 _ _ _] -> _
          tunnel: w197 -> [w212 w216 w219 w228 w242 w248 w254 w262 w273 _]
          tunnel: [w211 w215 w220 w229 w246 w252 w258 w261 w272 w275] -> w196
          tunnel: [w210 w213 w221 w230 w247 w253 w259 w260 w270 w276] -> w195
          tunnel: w194 -> [w210 w213 w221 w230 w247 w253 w259 w260 w270 w276]
          event Timeout {
            n104 = event-data() -> ()  [unwired: 1 in, 3 out]
            n105 = global read "国弘过程全局变量.vi" "DO"() -> (w198:T2)
            n106 = Unbundle By Name(w198) -> ("溶解氧电极零点"=→"电极零点":sgl, "溶解氧电极斜率"=→"电极斜率":sgl, "大气压补偿值"=→"气压补偿值":sgl, "盐度补偿值"=→"盐度补偿值":sgl, "溶解氧偏移修正值"=→"偏移值补偿":sgl, "溶解氧饱和度值"=→"饱和度值":sgl, "溶解氧测量值"=→"测量读值":sgl)  [unwired: 1 out]
            n107 = global read "多参数全局变量.vi" "DO通讯状态"() -> (w209:bool)
            n108 = property on="通讯状态" class="Str"("Blinking"=TRUE ("闪烁"), "Text.BG Color"=u32 16711680, "Visible"=w209) -> ()  [unwired: 2 in, 2 out]
            n109 = call "Add State to Queue.vi"("State(s) In (\"\")"=w212) -> ("States Out"=w211:string)  [unwired: 14 in]
            "通讯状态" <- "通讯异常" ("当前串口")
          }
          event "校准模式": Value Change {
            n110 = event-data() -> ()  [unwired: 1 in, 6 out]
            n111 = call "Add State to Queue.vi"("State(s) In (\"\")"=w216, "State(s) At Back (\"\")"="init: all\nidle" ("State(s) In (\"\")")) -> ("States Out"=w215:string)  [unwired: 13 in]
          }
          event "气压补偿值", "偏移值补偿": Mouse Down {
            n112 = event-data() -> ("CtlRef"=w218:refnum<vi>)  [unwired: 1 in, 7 out]
            n113 = property class="DigNum (严格)"(reference=w218) -> ("DisabledEnum"=w217:T3)  [unwired: 1 in, 2 out]
            n114 = case shown="\"Enabled\"" w217 {
              tunnel: w218 -> [w225 _]
              frame "Enabled" {
                n115 = property class="DigNum (严格)"(reference=w225) -> (reference out=w222:refnum<vi>, "Value"=w223:dbl)  [unwired: 1 in, 1 out]
                n116 = call "数字键盘.vi"("OldNumber"=w223) -> ("NewNumber"=w224:dbl)  [unwired: 1 in]
                n117 = property class="DigNum (严格)"(reference=w222, "Val(Sgnl)"=w224) -> ()  [unwired: 1 in, 2 out]
              }
              frame "Disabled", Default {
              }
            }
            n118 = call "Add State to Queue.vi"("State(s) In (\"\")"=w219) -> ("States Out"=w220:string)  [unwired: 14 in]
          }
          event "盐度补偿值": Mouse Down {
            n119 = event-data() -> ("CtlRef"=w227:refnum<vi>)  [unwired: 1 in, 7 out]
            n120 = property class="DigNum (严格)"(reference=w227) -> ("DisabledEnum"=w226:T3)  [unwired: 1 in, 2 out]
            n121 = case shown="\"Enabled\"" w226 {
              tunnel: w227 -> [w239 _]
              frame "Enabled" {
                n122 = global read "断电保存变量.vi" "Cond"() -> (w231:bool)
                n123 = case shown="真" w231 {
                  tunnel: [_ w240] -> w236
                  frame False {
                  }
                  frame True {
                    n124 = Two Button Dialog(message="是否使用系统测试值自动补偿" ("消息")) -> (T button?=w240:bool)  [unwired: 2 in]
                  }
                }
                n125 = global read "多参数全局变量.vi" "盐度显示"() -> (w235:T6)
                n126 = Unbundle By Name(w235) -> ("测量值"=w234:sgl)
                n127 = property class="DigNum (严格)"(reference=w239) -> (reference out=w237:refnum<vi>, "Value"=w233:dbl)  [unwired: 1 in, 1 out]
                n128 = Select(t=w234, s=w236, f=w233) -> (s? t:f=w232:dbl)
                n129 = call "数字键盘.vi"("OldNumber"=w232) -> ("NewNumber"=w238:dbl)  [unwired: 1 in]
                n130 = property class="DigNum (严格)"(reference=w237, "Val(Sgnl)"=w238) -> ()  [unwired: 1 in, 2 out]
              }
              frame "Disabled", Default {
              }
            }
            n131 = call "Add State to Queue.vi"("State(s) In (\"\")"=w228) -> ("States Out"=w229:string)  [unwired: 14 in]
          }
          event "盐度补偿值": Value Change {
            n132 = event-data() -> ("NewVal"=w244:dbl)  [unwired: 1 in, 5 out]
            n133 = global read "多参数全局变量.vi" "MB session in"() -> (w245:refnum<class "MB_Master.lvclass">)
            n134 = call "0008H_DO_盐度补偿值写入.vi"("数值"=w244, "MB session in"=w245) -> ("error out"=w243:errorcluster)  [unwired: 8 in, 1 out]
            n135 = call "Add State to Queue.vi"("State(s) In (\"\")"=w242) -> ("States Out"=w246:string)  [unwired: 14 in]
          }
          event "气压补偿值": Value Change {
            n136 = event-data() -> ("NewVal"=w250:dbl)  [unwired: 1 in, 5 out]
            n137 = global read "多参数全局变量.vi" "MB session in"() -> (w251:refnum<class "MB_Master.lvclass">)
            n138 = call "000AH_DO_大气压补偿值写入.vi"("数值"=w250, "MB session in"=w251) -> ("error out"=w249:errorcluster)  [unwired: 8 in, 1 out]
            n139 = call "Add State to Queue.vi"("State(s) In (\"\")"=w248) -> ("States Out"=w252:string)  [unwired: 14 in]
          }
          event "偏移值补偿": Value Change {
            n140 = event-data() -> ("NewVal"=w256:dbl)  [unwired: 1 in, 5 out]
            n141 = global read "多参数全局变量.vi" "MB session in"() -> (w257:refnum<class "MB_Master.lvclass">)
            n142 = call "000CH_DO_DO偏移修正值写入.vi"("数值"=w256, "MB session in"=w257) -> ("error out"=w255:errorcluster)  [unwired: 8 in, 1 out]
            n143 = call "Add State to Queue.vi"("State(s) In (\"\")"=w254) -> ("States Out"=w258:string)  [unwired: 14 in]
          }
          event "刷新按钮": Value Change {
            n144 = event-data() -> ()  [unwired: 1 in, 6 out]
            n145 = call "Add State to Queue.vi"("State(s) In (\"\")"=w262) -> ("States Out"=w261:string)  [unwired: 14 in]
            n146 = Two Button Dialog(message="请再次确实是否恢复出厂设置！" ("消息")) -> (T button?=w264:bool)  [unwired: 2 in]
            n147 = case shown="真" w264 {
              frame False {
              }
              frame True {
                w265 = u16 33 items=["Factory Reset"=33] ("数值")
                n148 = global read "多参数全局变量.vi" "MB session in"() -> (w266:refnum<class "MB_Master.lvclass">)
                n149 = call "0026H_DO_命令寄存器写入.vi"("数值"=w265, "MB session in"=w266) -> ()  [unwired: 8 in, 2 out]
              }
            }
          }
          event "校准启动": Value Change {
            n150 = event-data() -> ()  [unwired: 1 in, 6 out]
            n151 = global read "多参数全局变量.vi" "校准运行状态"() -> (w268:T5)
            n152 = call "Add State to Queue.vi"("State(s) In (\"\")"=w273, "State(s) At Back (\"\")"="init: all\nCal: Place standard solution\n Cal: Calibration process\nidle" ("State(s) In (\"\")")) -> ("States Out"=w272:string)  [unwired: 13 in]
            n153 = Bundle By Name(cluster=w268, "DO"=TRUE) -> (w269:T5)
            n154 = global write "多参数全局变量.vi" "校准运行状态"(w269) -> ()
          }
          event "校准停止": Value Change {
            n155 = event-data() -> ()  [unwired: 1 in, 6 out]
            n156 = call "Add State to Queue.vi"("State(s) In (\"\")"="init: all\nCal: Over\nidle" ("State(s) In (\"\")")) -> ("States Out"=w275:string)  [unwired: 14 in]
          }
        }
      }
    }
  }
  n157 = while {
    stop <- FALSE stop-if-true
    n158 = global read "多参数全局变量.vi" "权限"() -> (w280:enum16{"一级权限", "二级权限", "三级权限"})
    n159 = Wait (ms)(milliseconds to wait=u32 1000 ("等待时间（毫秒）")) -> ()  [unwired: 1 out]
    n160 = Not Equal?(x=w280, y=enum16{"一级权限", "二级权限", "三级权限"}."一级权限") -> (x != y?=w278:bool)
    n161 = property on="偏移值补偿" class="DigNum (严格)"("Visible"=w278) -> ()  [unwired: 2 in, 2 out]
  }
